vi "ATS_GetBoardBySystemId.vi"(7 "Sys/Board_In":T1) -> (2 "Handle":u32, 3 "Sys/Board_Out":T1)   [LabVIEW 2010]
doc: "_____AlazarTech, Scope_____\n\nRetrieve the handle for a given device.\n\nInput: \nSys/Board_In:\n \"System\" = system identification number. Must be >0.\n \"Board\" = board identification number in the system. Must be >0.\n\nOutput:\nSys/Board_Out: duplicate Sys/Board_In\n\"Handle\" = handle of the selected board\n\nA System can be one board or many board in a master slave configuration.\nIn master/slave configuration the System indicate the group starting at 1 and the Board select the device in that group of board starting at 1 up to the number of board in the system..\nIf multi board are in one computer (not in master/slave configuration) then the identification for each board will be:\n System = id of the board starting at 1 up to number of board in the computer and Board=1."
uses:
  ATS_ctl/ATS_Sys_Board.ctl
  ATSApi.dll
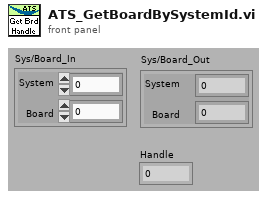
[diagram p1: front panel]
types:
  T1 = typedef "ATS_Sys_Board.ctl" = cluster{"System":u32, "Board":u32}
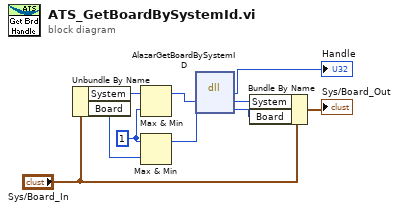
[diagram p0: block diagram]
diagram:
  w10 = u32 1 ("y")
  n1 = Unbundle By Name("Sys/Board_In") -> ("System"=w3:u32, "Board"=w4:u32)
  n2 = Max & Min(x=w3, y=w10) -> (max(x,y)=w7:u32)  [unwired: 1 out]
  n3 = Max & Min(x=w10, y=w4) -> (max(x,y)=w9:u32)  [unwired: 1 out]
  n4 = dll-call lib="ATSApi.dll" fn="AlazarGetBoardBySystemID"("sid"=w7, "brdNum"=w9) -> (→"Handle":u32, "sid"=w1:u32, "brdNum"=w2:u32)  [unwired: 3 in, 2 out]
  n5 = Bundle By Name(cluster="Sys/Board_In", "System"=w1, "Board"=w2) -> (→"Sys/Board_Out":T1)
